vi "Write AutoSizeRowsMode.vi"(8 "error in (no error)":errorcluster, 10 "AutoSizeRowsMode":i32(ring)=11 items=["None"=0, "AllHeaders"=5, "AllCellsExceptHeaders"=6, "AllCells"=7, "DisplayedHeaders"=9, "DisplayedCellsExceptHeaders"=10, "DisplayedCells"=11], 11 "DataGridView in":refnum<class "DataGridView.lvclass">) -> (0 "error out":errorcluster, 3 "DataGridView out":refnum<class "DataGridView.lvclass">)   [LabVIEW 2014, in "DataGridView.lvclass"]
uses:
  DataGridView.lvclass
  DataGridView.lvclass/DataGridView.ctl
  System.Windows.Forms
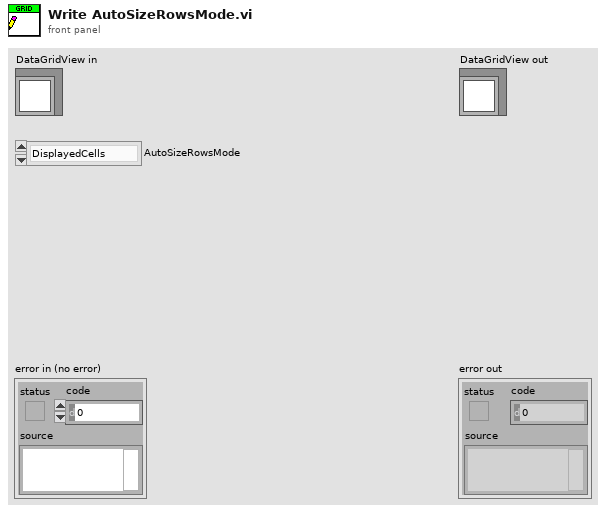
[diagram p1: front panel]
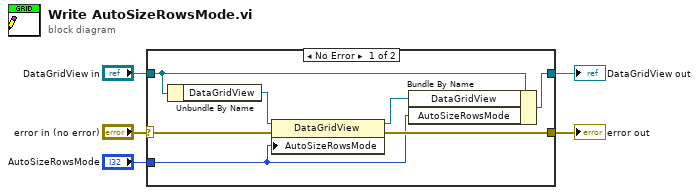
[diagram p0: block diagram]
diagram:
  n1 = case shown="No Error" "error in (no error)" {
    selector: "error in (no error)" -> [w8 w13]
    tunnel: [w7 w13] -> w4
    tunnel: [w12 w14] -> w2
    tunnel: "DataGridView in" -> [w11 w14]
    tunnel: "AutoSizeRowsMode" -> [w6 _]
    frame No Error {
      n2 = Unbundle By Name(w11) -> ("DataGridView"=w10:refnum<k24>)
      n3 = property class="DataGridView"(reference=w10, error in=w8, "AutoSizeRowsMode"=w6) -> (reference out=w9:refnum<k24>, error out=w7:errorcluster)
      n4 = Bundle By Name(cluster=w11, "DataGridView"=w9, "AutoSizeRowsMode"=w6) -> (w12:refnum<class "DataGridView.lvclass">)
    }
    frame Error {
    }
  }
  "error out" <- w4
  "DataGridView out" <- w2
